vi "MoveSelection.vi"(8 "error in (no error)":errorcluster, 9 "down?":bool, 10 "up?":bool, 11 "Cursor in":refnum<class "Cursor.lvclass">) -> (0 "error out":errorcluster, 3 "Cursor out":refnum<class "Cursor.lvclass">)   [LabVIEW 2019, in "RT_Game.lvlib" / "Cursor.lvclass"]
uses:
  Cursor.lvclass
  C:/Users/FreshBob/Dropbox/VIs/myRIO_GameConsole/RT/RT_Game/GameObject/GameObject.lvclass
  Cursor.lvclass/Cursor.ctl
  GameObject/GameObject.lvclass
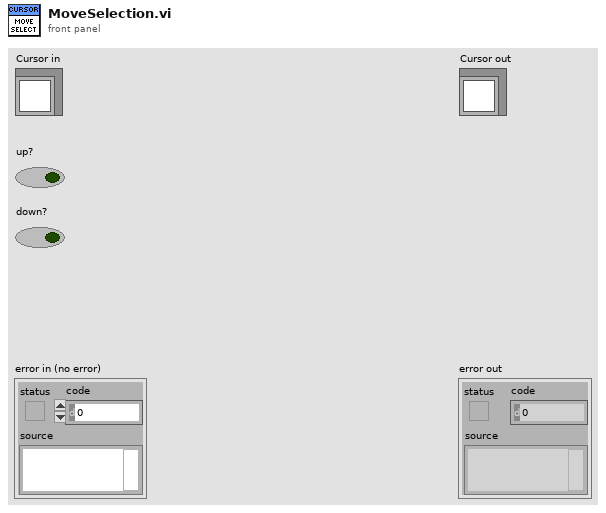
[diagram p1: front panel]
types:
  T1 = typedef "RT_Game.lvlib/Game.lvclass/Coordinate.ctl" = cluster{"x":dbl, "y":dbl}
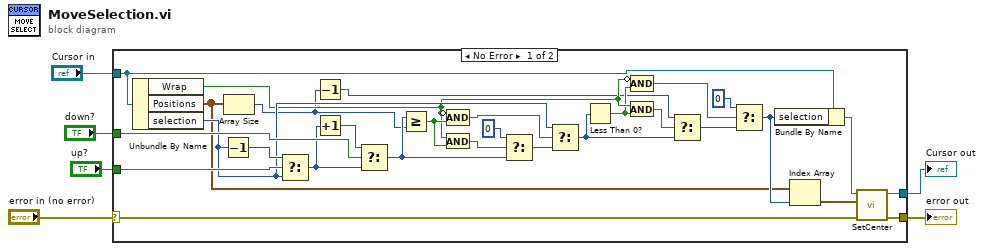
[diagram p0: block diagram]
diagram:
  n1 = case shown="No Error" "error in (no error)" {
    selector: "error in (no error)" -> [w35 w37]
    tunnel: [w12 w37] -> w5
    tunnel: [w10 w36] -> w3
    tunnel: "Cursor in" -> [w34 w36]
    tunnel: "up?" -> [w33 _]
    tunnel: "down?" -> [w32 _]
    frame No Error {
      n2 = Unbundle By Name(w34) -> ("Wrap"=w19:bool, "Positions"=w8:T1[], "selection"=w22:i16)
      n3 = Decrement(x=w22) -> (x-1=w31:i16)
      n4 = Array Size(array=w8) -> (size(s)=w16:i32)
      n5 = Select(t=w31, s=w33, f=w22) -> (s? t:f=w30:i16)
      n6 = Decrement(x=w16) -> (x-1=w15:i32)
      n7 = Increment(x=w30) -> (x+1=w29:i16)
      n8 = Select(t=w29, s=w32, f=w30) -> (s? t:f=w28:i16)
      n9 = Greater Or Equal?(x=w28, y=w16) -> (x >= y?=w24:bool)
      n10 = And(x=w19, y=w24) -> (x .and. y?=w26:bool)
      n11 = Compound Arithmetic op=AND(invert w19, w24) -> (w23:bool)
      n12 = Select(t=i16 0, s=w26, f=w28) -> (s? t:f=w27:i16)
      n13 = Select(t=w22, s=w23, f=w27) -> (s? t:f=w21:i16)
      n14 = Less Than 0?(x=w21) -> (x < 0?=w18:bool)
      n15 = And(x=w19, y=w18) -> (x .and. y?=w17:bool)
      n16 = Compound Arithmetic op=AND(invert w19, w18) -> (w14:bool)
      n17 = Select(t=w15, s=w17, f=w21) -> (s? t:f=w20:i32)
      n18 = Select(t=0, s=w14, f=w20) -> (s? t:f=w9:i32)
      n19 = Bundle By Name(cluster=w34, "selection"=w9) -> (w11:refnum<class "Cursor.lvclass">)
      n20 = Index Array(array=w8, index=w9) -> (element=w7:T1)
      n21 = call "SetCenter.vi"("error in (no error)"=w35, "center_position"=w7, "GameObject in"=w11) -> ("error out"=w12:errorcluster, "GameObject out"=w10:refnum<class "Cursor.lvclass">)  [unwired: 7 in]
    }
    frame Error {
    }
  }
  "error out" <- w5
  "Cursor out" <- w3
